vi "Change Mode - Speed Control.vi"(3 "D":dbl, 4 "I":dbl, 5 "P":dbl, 6 "CAN Jaguar Ref":T1={"DeviceStatus"={"status"=FALSE, "code"=0, "source"=""}, "Type"=enum."PWM", "PWM"={"Digital Module"=enum."Digital Module 2", "PWM Channel"=enum."PWM 1", "DeadBand"={"Name"="", "maxPositivePwm"=0, "minPositivePwm"=0, "centerPwm"=0, "maxNegativePwm"=0, "minNegativePwm"=0, "angularRange"=0}}, "CAN"={"Device Number"=0, "Control Mode"=enum."Percent VBus", "Semaphore"=refnum, "Max Vout"=12.0}, "Invert"=FALSE, "TransformRef"=refnum, "InvTransformRef"=refnum}) -> ()   [LabVIEW 2011]
uses:
  <vilib>/Rock Robotics/WPI/MotorControl/WPI_MotorControlDeviceRef.ctl
  <vilib>/Rock Robotics/SystemInterfaces/Typedef/FPGA_TypedefDigitalModule.ctl
  <vilib>/Rock Robotics/SystemInterfaces/DIO/FPGA_DIOPWMChannel.ctl
  <vilib>/Rock Robotics/WPI/PWM/WPI_PWMDeadband.ctl
  <vilib>/Rock Robotics/WPI/CAN/Jaguar/SubVIs/WPI_CANJaguar_ControlMode.ctl
  <vilib>/Rock Robotics/WPI/PWM/WPI_PWMTransform_ConPane.ctl
  <vilib>/Rock Robotics/WPI/CAN/Jaguar/SubVIs/WPI_CANJaguar_SpeedReference.ctl
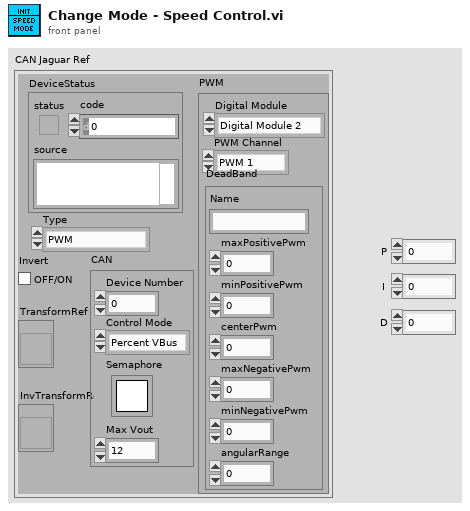
[diagram p1: front panel]
types:
  T1 = typedef "WPI_MotorControlDeviceRef.ctl" = cluster{"DeviceStatus":errorcluster, "Type":enum16{"PWM", "CAN"}, "PWM":cluster{"Digital Module":T2, "PWM Channel":T3, "DeadBand":T4}, "CAN":cluster{"Device Number":u8, "Control Mode":T5, "Semaphore":T6, "Max Vout":dbl}, "Invert":bool, "TransformRef":T7, "InvTransformRef":T7}
  T2 = typedef "FPGA_TypedefDigitalModule.ctl" = enum16{"Digital Module 1", "Digital Module 2"}
  T3 = typedef "FPGA_DIOPWMChannel.ctl" = enum8{"PWM 1", "PWM 2", "PWM 3", "PWM 4", "PWM 5", "PWM 6", "PWM 7", "PWM 8", "PWM 9", "PWM 10", "Invalid"}
  T4 = typedef "WPI_PWMDeadband.ctl" = cluster{"Name":string, "maxPositivePwm":i32, "minPositivePwm":i32, "centerPwm":i32, "maxNegativePwm":i32, "minNegativePwm":i32, "angularRange":u16}
  T5 = typedef "WPI_CANJaguar_ControlMode.ctl" = enum8{"Percent VBus", "Current", "Speed", "Position", "Voltage"}
  T6 = typedef "Semaphore RefNum" = refnum<k1>
  T7 = typedef "WPI_PWMTransform_ConPane.ctl" = refnum<vi>
  T8 = typedef "WPI_CANJaguar_SpeedReference.ctl" = u8
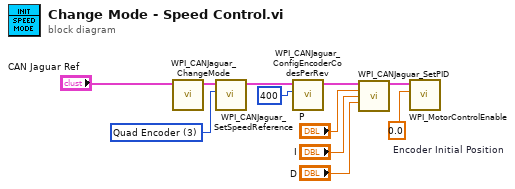
[diagram p0: block diagram]
diagram:
  w2 = T8 3 items=["Encoder"=0, "Inv Encoder"=2, "Quad Encoder"=3, "None"=255] ("Speed Reference")
  w11 = 0.0  # Encoder Initial Position
  n1 = call <vilib>:"WPI_CANJaguar_ChangeMode.vi"("CAN Jaguar Ref"="CAN Jaguar Ref") -> ("CAN Jaguar Ref Out"=w3:T1)  [unwired: 9 in, 1 out]
  n2 = call <vilib>:"WPI_CANJaguar_SetSpeedReference.vi"("Speed Reference"=w2, "CAN Jaguar Ref"=w3) -> ("CAN Jaguar Ref Out"=w10:T1)  [unwired: 8 in, 1 out]
  n3 = call <vilib>:"WPI_CANJaguar_ConfigEncoderCodesPerRev.vi"("Encoder Codes Per Rev"=u16 400, "CAN Jaguar Ref"=w10) -> ("CAN Jaguar Ref Out"=w8:T1)  [unwired: 8 in, 1 out]
  n4 = call <vilib>:"WPI_CANJaguar_SetPID.vi"("CAN Jaguar Ref"=w8, "P"="P", "I"="I", "D"="D") -> ("CAN Jaguar Ref Out"=w4:T1)  [unwired: 10 in, 1 out]
  n5 = call <vilib>:"WPI_MotorControlEnable.vi"("Encoder Initial Position"=w11, "CAN Jaguar Ref"=w4) -> ()  [unwired: 8 in, 2 out]
